vi "BAM Generation Search for Connection (Local Message).vi"(0 "Connections":T2[](array[typedef]) {"Packets"."Identifier" format="%08x"}, 5 "Data to Send":T1 {"Identifier" format="%08x"}, 11 "error in (no error)":errorcluster) -> (4 "Connection Cluster":T2 {"Packets"."Identifier" format="%08x"}, 6 "CAN Frame Out":T1 {"Identifier" format="%08x"}, 8 "Found?":bool, 10 "Index":i32, 15 "error out":errorcluster)   [LabVIEW 2015, in "J1939 Addon Engine.lvlib"]
uses:
  Engine/J1939 Addon Engine.lvlib
  Types/BAM Generation Connection Cluster.ctl
  J1939 Utilities/Types/CAN Outgoing Message Cluster.ctl
  J1939 Utilities/SubVIs/Convert CAN Arb ID to J1939 ID.vi
  J1939 Utilities/J1939 Utilities.lvlib
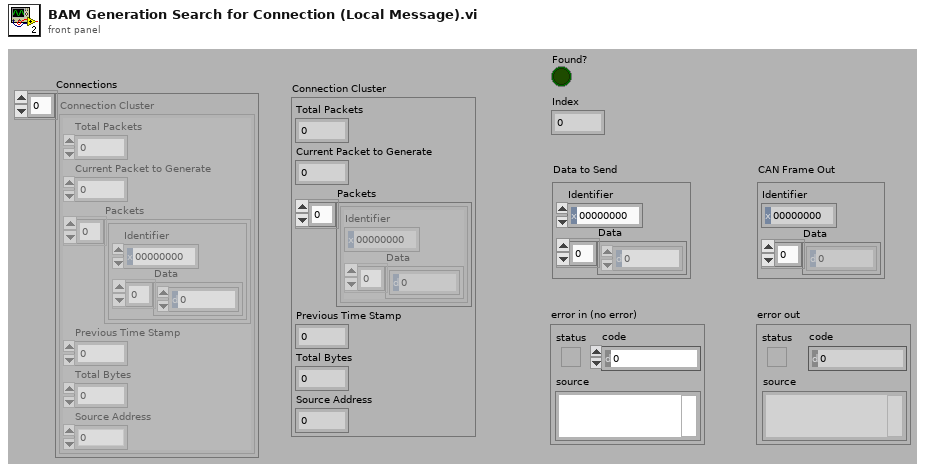
[diagram p1: front panel]
types:
  T1 = typedef "J1939 Addon Shared.lvlib/J1939 Utilities.lvlib/CAN Outgoing Message Cluster.ctl" = cluster{"Identifier":u32, "Data":u8[]}
  T2 = typedef "J1939 Addon Engine.lvlib/BAM Generation Connection Cluster.ctl" = cluster{"Total Packets":u8, "Current Packet to Generate":u8, "Packets":T1[], "Previous Time Stamp":u32, "Total Bytes":u16, "Source Address":u8}
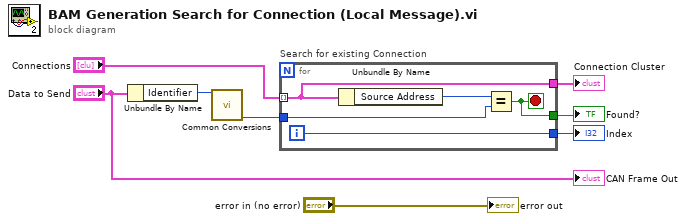
[diagram p0: block diagram]
diagram:
  n1 = Unbundle By Name("Data to Send") -> ("Identifier"=w2:u32)
  n2 = call-poly "Common Conversions.vi"("Arb ID"=w2) -> ("Source Address"=w1:u8)  [unwired: 14 out]
  n3 = for "Search for existing Connection" {
    tunnel: "Connections" -> [w9] mode=indexing
    tunnel: [w12] -> w6
    tunnel: w1 -> [w11]
    tunnel: [w10] -> w5
    tunnel: [w9] -> w7
    i -> [w10]
    stop <- w12 stop-if-true
    n4 = Unbundle By Name(w9) -> ("Source Address"=w13:u8)
    n5 = Equal?(x=w13, y=w11) -> (x = y?=w12:bool)
  }
  "Connection Cluster" <- w7
  "Found?" <- w6
  "Index" <- w5
  "error out" <- "error in (no error)"
  "CAN Frame Out" <- "Data to Send"
